vi "IVC_read.vi"(8 "error in (no error)":errorcluster, 11 "VISA Refnum in":refnum<visa-resource-name>="COM7") -> (0 "error out":errorcluster, 1 "read buffer":string, 2 "IVC":string, 3 "VISA Refnum out":refnum<visa-resource-name>, 4 "return count":u32, 5 "concatenated string":string)   [LabVIEW 2019]
panel:
  out "concatenated string 3":string
  out "concatenated string 2":string
  out "VISA resource name out":refnum<visa-resource-name>
  in  "Numeric":dbl
  in  "channel 2":string="0320074002=?"
  in  "channel 1":string="0320074002=?"
  out "substring":string
  out "x-y*floor(x/y)":u64
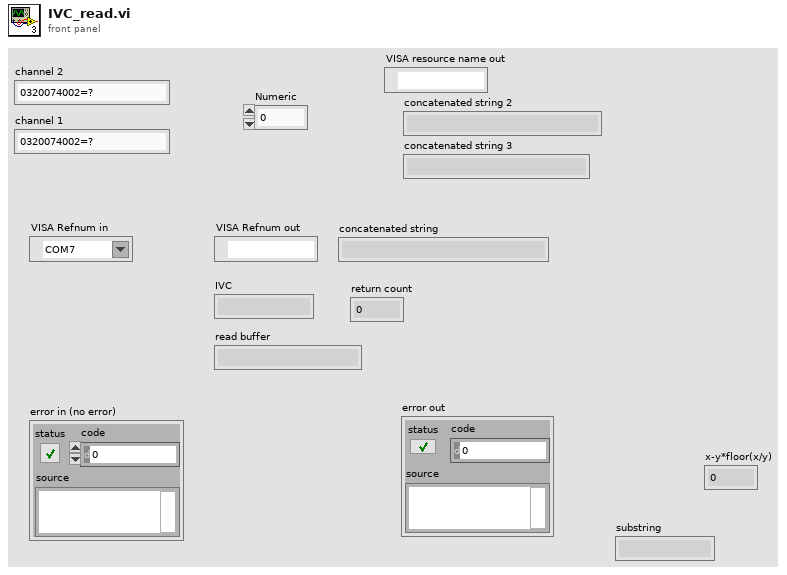
[diagram p1: front panel]
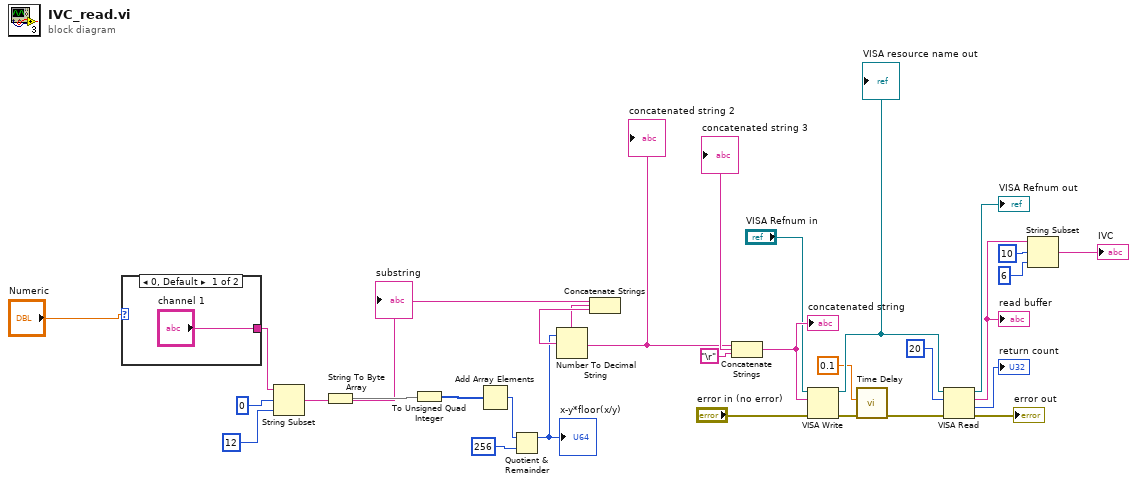
[diagram p0: block diagram]
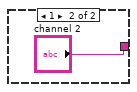
[diagram p2: hidden frame]
diagram:
  n1 = case shown="0, Default" "Numeric" {
    tunnel: ["channel 1" "channel 2"] -> w1
    frame 0, Default {
    }
    frame 1 {
    }
  }
  n2 = String Subset(string=w1, offset (0)=0, length (rest)=12 ("length (rest)")) -> (substring=w6:string)
  "substring" <- w6
  n3 = String To Byte Array(string=w6) -> (unsigned byte array=w9:u8[])
  n4 = To Unsigned Quad Integer(1:w9) -> (0:w10:u64[])
  n5 = Add Array Elements(numeric array=w10) -> (sum=w8:u64)
  n6 = Quotient & Remainder(x=w8, y=u64 256) -> (x-y*floor(x/y)=w4:u64)  [unwired: 1 out]
  "x-y*floor(x/y)" <- w4
  n7 = Number To Decimal String(number=w4) -> (decimal integer string=w5:string)  [unwired: 1 in]
  n8 = Concatenate Strings(w6, w5) -> (w3:string)
  "concatenated string 2" <- w3
  n9 = Concatenate Strings(w3, "\r") -> (w22:string)
  "concatenated string" <- w22
  "concatenated string 3" <- w22
  n10 = VISA Write(VISA resource name="VISA Refnum in", write buffer=w22, error in (no error)="error in (no error)") -> (VISA resource name out=w19:refnum<visa-resource-name>, error out=w21:errorcluster)  [unwired: 1 out]
  "VISA resource name out" <- w19
  n11 = call "Time Delay"("error in (no error)"=w21, "Delay Time (s)"=0.1) -> ("error out"=w16:errorcluster)  [unwired: 9 in]
  n12 = VISA Read(VISA resource name=w19, byte count=u32 20, error in (no error)=w16) -> (VISA resource name out=→"VISA Refnum out":refnum<visa-resource-name>, read buffer=w27:string, return count=→"return count":u32, error out=→"error out":errorcluster)
  "read buffer" <- w27
  n13 = String Subset(string=w27, offset (0)=10, length (rest)=6 ("length (rest)")) -> (substring=→"IVC":string)
